vi "Write Strings And Values [].vi"(5 "Strings And Values []":cluster{"String":string, "Value":variant}[](array[cluster]), 9 "Ring in":refnum<class "Ring.lvclass">) -> (3 "Ring out":refnum<class "Ring.lvclass">)   [LabVIEW 2014, in "Ring.lvclass"]
uses:
  Ring.lvclass
  Ring.lvclass/Ring.ctl
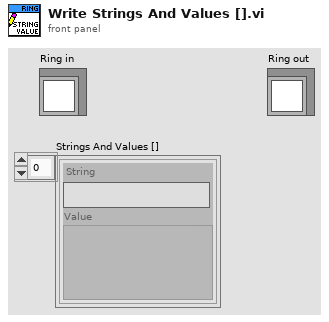
[diagram p1: front panel]
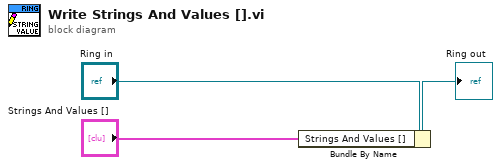
[diagram p0: block diagram]
diagram:
  n1 = Bundle By Name(cluster="Ring in", "Strings And Values []"="Strings And Values []") -> (→"Ring out":refnum<class "Ring.lvclass">)
